vi "Request Data JSON.vi"(8 "error in (no error)":errorcluster, 11 "GetSceneItemID in":refnum<class "GetSceneItemID.lvclass">) -> (0 "error out":errorcluster, 2 "Request Data JSON":string, 3 "GetSceneItemID out":refnum<class "GetSceneItemID.lvclass">)   [LabVIEW 2020, in "obs-websocket.lvlib" / "GetSceneItemID.lvclass"]
uses:
  GetSceneItemID.lvclass
  GetSceneItemID.lvclass/GetSceneItemID.ctl
  3dafc9c7-2ee4-40f4-92d1-9f060d7c6dc8.vi
  <vilib>/JDP Science/JSONtext/Variant to JSON Text.vi
  <vilib>/JDP Science/JSONtext/LVClass Serializer/JSONtext LVClass Serializer.lvclass
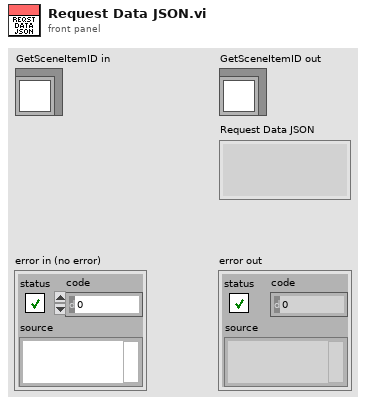
[diagram p1: front panel]
types:
  T1 = cluster{"sceneName":string, "sourceName":string, "searchOffset":i32}
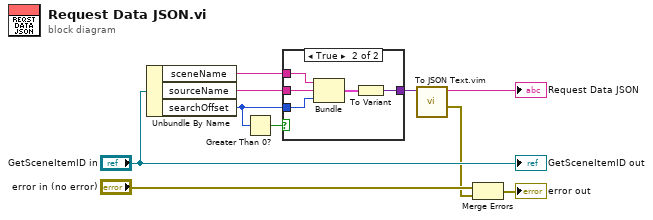
[diagram p0: block diagram]
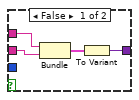
[diagram p2: hidden frame]
diagram:
  n1 = Unbundle By Name("GetSceneItemID in") -> ("sceneName"=w5:string, "sourceName"=w6:string, "searchOffset"=w8:i32)
  n2 = Greater Than 0?(x=w8) -> (x > 0?=w7:bool)
  n3 = case shown="True" w7 {
    tunnel: w8 -> [_ w17]
    tunnel: w6 -> [w14 w19]
    tunnel: w5 -> [w13 w18]
    tunnel: [w11 w15] -> w4
    frame False {
      n4 = Bundle("sceneName"=w13, "sourceName"=w14) -> (w12:cluster{"sceneName":string, "sourceName":string})  [unwired: 1 in]
      n5 = To Variant(anything=w12) -> (Variant=w11:variant)
    }
    frame True {
      n6 = Bundle("sceneName"=w18, "sourceName"=w19, "searchOffset"=w17) -> (w16:T1)  [unwired: 1 in]
      n7 = To Variant(anything=w16) -> (Variant=w15:variant)
    }
  }
  n8 = call "To JSON Text.vim"("Anything"=w4) -> ("error out"=w2:errorcluster, "<JSON>"=→"Request Data JSON":string)  [unwired: 9 in]
  n9 = Merge Errors("error in (no error)", w2) -> (→"error out":errorcluster)
  "GetSceneItemID out" <- "GetSceneItemID in"
